vi "Pelletron_Conditioning.vi"(6 "Desired Voltage (MV)":dbl, 7 "Condition Start time":dbl, 8 "error in (no error)":errorcluster, 9 "Input Old Cluster":T1, 10 "Input New Cluster":T2, 11 "AccelNET.lvlib:TCP.lvclass":refnum<class "TCP.lvclass">) -> (0 "Error Out":errorcluster, 1 "Conditioning?":bool, 2 "Step Up Voltage?":bool)   [LabVIEW 2012, in "AccelNET.lvlib" / "TCP.lvclass"]
uses:
  TCP.lvclass
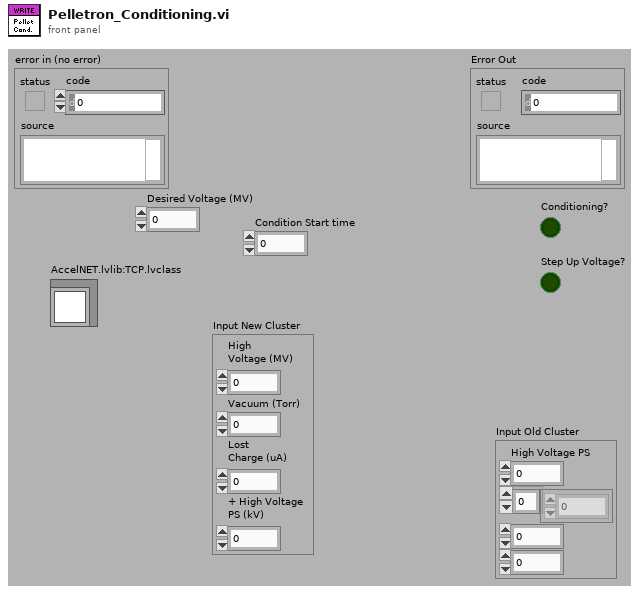
[diagram p1: front panel]
types:
  T1 = cluster{"High Voltage PS":dbl, "Pressure":dbl[], "Lost Charge":dbl, "High Voltage":dbl}
  T2 = cluster{"High\nVoltage (MV)":dbl, "Vacuum (Torr)":dbl, "Lost\nCharge (uA)":dbl, "+ High Voltage\nPS (kV)":dbl}
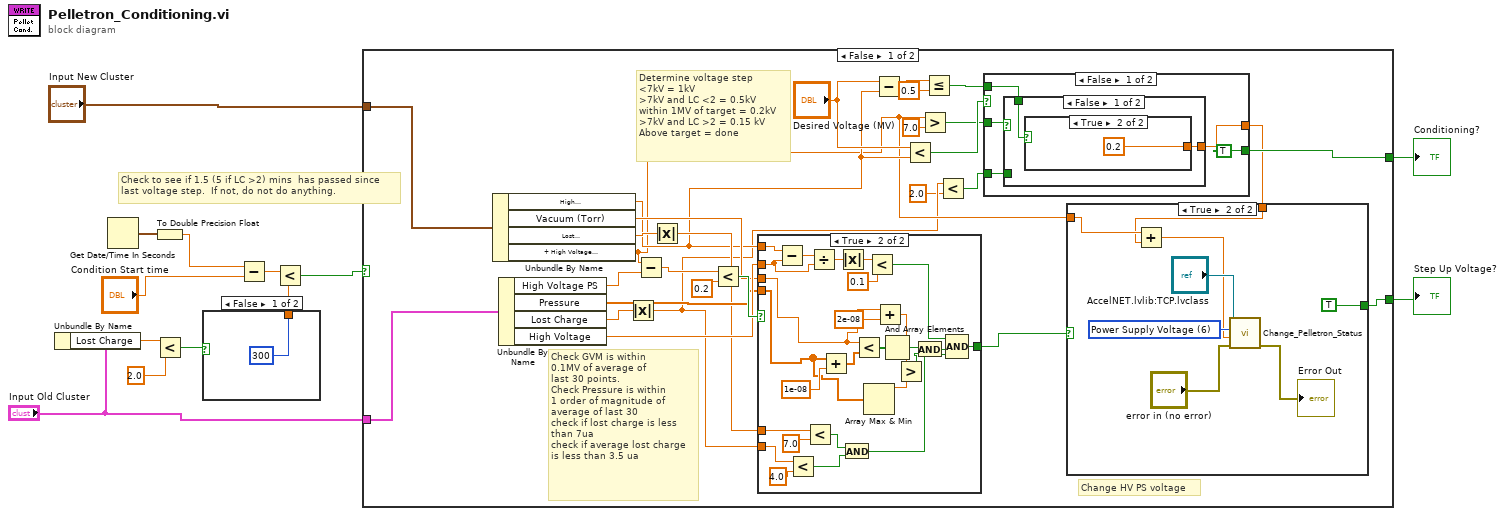
[diagram p0: block diagram]
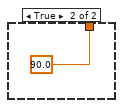
[diagram p2: hidden frame]
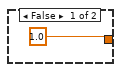
[diagram p3: hidden frame]
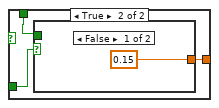
[diagram p4: hidden frame]
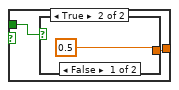
[diagram p5: hidden frame]
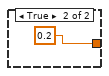
[diagram p6: hidden frame]
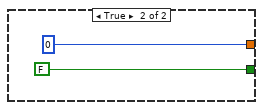
[diagram p7: hidden frame]
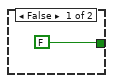
[diagram p8: hidden frame]
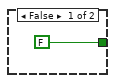
[diagram p9: hidden frame]
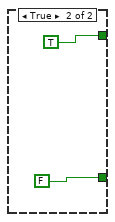
[diagram p10: hidden frame]
diagram:
  # "Check to see if 1.5 (5 if LC >2) mins  has passed since\nlast voltage step.  If not, do not do anything."
  n1 = Unbundle By Name("Input Old Cluster") -> ("Lost Charge"=w3:dbl)
  n2 = Get Date/Time In Seconds() -> (seconds since 1Jan1904=w13:timestamp)
  n3 = To Double Precision Float(number=w13) -> (double precision float=w12:dbl)
  n4 = Less?(x=w3, y=2.0) -> (x < y?=w1:bool)
  n5 = case shown="False" w1 {
    tunnel: [300 90.0 ("y")] -> w9
    frame False {
    }
    frame True {
    }
  }
  n6 = Subtract(x=w12, y="Condition Start time") -> (x-y=w10:dbl)
  n7 = Less?(x=w10, y=w9) -> (x < y?=w8:bool)
  n8 = case shown="False" w8 {
    tunnel: [w28 FALSE] -> w7
    tunnel: [w27 TRUE] -> w6
    tunnel: "Input New Cluster" -> [w20 _]
    tunnel: "Input Old Cluster" -> [w19 _]
    frame False {
      # "Change HV PS voltage"
      # "Determine voltage step\n<7kV = 1kV\n>7kV and LC <2 = 0.5kV\nwithin 1MV of target = 0.2kV\n>7kV and LC >2 = 0.15 kV\nAbove target = done"
      # "Check GVM is within\n0.1MV of average of\nlast 30 points.\nCheck Pressure is within\n1 order of magnitude of\naverage of last 30\ncheck if lost charge is less\nthan 7ua\ncheck if average lost charge\nis less than 3.5 ua"
      n9 = Unbundle By Name(w20) -> ("High\nVoltage (MV)"=w26:dbl, "Vacuum (Torr)"=w39:dbl, "Lost\nCharge (uA)"=w37:dbl, "+ High Voltage\nPS (kV)"=w21:dbl)
      n10 = Unbundle By Name(w19) -> ("High Voltage PS"=w43:dbl, "Pressure"=w38:dbl[], "Lost Charge"=w36:dbl, "High Voltage"=w40:dbl)
      n11 = Absolute Value(x=w36) -> (abs(x)=w18:dbl)
      n12 = Subtract(x=w21, y=w43) -> (x-y=w22:dbl)
      n13 = Absolute Value(x=w37) -> (abs(x)=w35:dbl)
      n14 = Less?(x=w22, y=0.2) -> (x < y?=w41:bool)
      n15 = case shown="True" w41 {
        tunnel: w26 -> [_ w94]
        tunnel: w40 -> [_ w92]
        tunnel: w39 -> [_ w76]
        tunnel: w38 -> [_ w80]
        tunnel: w35 -> [_ w98]
        tunnel: w18 -> [_ w96]
        tunnel: [FALSE w85] -> w23
        frame False {
        }
        frame True {
          n16 = Subtract(x=w94, y=w92) -> (x-y=w93:dbl)
          n17 = Less?(x=w96, y=4.0) -> (x < y?=w88:bool)
          n18 = Less?(x=w98, y=7.0) -> (x < y?=w89:bool)
          n19 = Divide(x=w93, y=w92) -> (x/y=w91:dbl)
          n20 = Add(x=w80, y=1e-08) -> (x+y=w81:dbl[])
          n21 = Absolute Value(x=w91) -> (abs(x)=w83:dbl)
          n22 = And(x=w89, y=w88) -> (x .and. y?=w86:bool)
          n23 = Less?(x=w76, y=w81) -> (x < y?=w84:bool[])
          n24 = Array Max & Min(array=w80) -> (max value=w78:dbl)  [unwired: 3 out]
          n25 = Less?(x=w83, y=0.1) -> (x < y?=w87:bool)
          n26 = Add(x=w76, y=2e-08) -> (x+y=w74:dbl)
          n27 = And Array Elements(Boolean array=w84) -> (logical AND=w79:bool)
          n28 = Greater?(x=w74, y=w78) -> (0:w77:bool)
          n29 = And(x=w79, y=w77) -> (x .and. y?=w73:bool)
          n30 = Compound Arithmetic op=AND(w87, w73, w86) -> (w85:bool)
        }
      }
      n31 = Subtract(x="Desired Voltage (MV)", y=w26) -> (x-y=w33:dbl)
      n32 = Less?(x="Desired Voltage (MV)", y=w26) -> (x < y?=w30:bool)
      n33 = Greater?(x=w21, y=7.0) -> (0:w25:bool)
      n34 = Less Or Equal?(x=w33, y=0.5) -> (x <= y?=w29:bool)
      n35 = Less?(x=w18, y=2.0) -> (x < y?=w16:bool)
      n36 = case shown="False" w30 {
        tunnel: [TRUE FALSE] -> w27
        tunnel: [w45 0] -> w24
        tunnel: w29 -> [w47 _]
        tunnel: w25 -> [w48 _]
        tunnel: w16 -> [w44 _]
        frame False {
          n37 = case shown="False" w48 {
            tunnel: w47 -> [w50 w55]
            tunnel: [w49 w54] -> w45
            tunnel: w44 -> [_ w53]
            frame False {
              n38 = case shown="True" w50 {
                tunnel: [1.0 ("y") 0.2 ("y")] -> w49
                frame False {
                }
                frame True {
                }
              }
            }
            frame True {
              n39 = case shown="False" w53 {
                tunnel: w55 -> [_ w58]
                tunnel: [0.15 w57] -> w54
                frame False {
                }
                frame True {
                  n40 = case shown="False" w58 {
                    tunnel: [0.5 ("y") 0.2 ("y")] -> w57
                    frame False {
                    }
                    frame True {
                    }
                  }
                }
              }
            }
          }
        }
        frame True {
        }
      }
      n41 = case shown="True" w23 {
        tunnel: [FALSE TRUE] -> w28
        tunnel: w24 -> [_ w65]
        tunnel: w21 -> [_ w66]
        frame False {
        }
        frame True {
          w71 = u16 6 items=["GV", "Blower", "Main Power Supply", "Chain Power Supply", "Chain", "Rotating Shaft", "Power Supply Voltage", "Control Mode", "Control Mode Reference", "Chain Bypass", "Rotating Shaft Bypass", "Spark Counter", "Spark Limit", "Threshold", "Spark Counter Reset", "Ion Filament"] ("Write Selector")
          n42 = Add(x=w66, y=w65) -> (x+y=w64:dbl)
          n43 = call "Change_Pelletron_Status.vi"("error in (no error)"="error in (no error)", "Write Value"=w64, "Write Selector"=w71, "AccelNET.lvlib:TCP.lvclass"="AccelNET.lvlib:TCP.lvclass") -> ("error out"=→"Error Out":errorcluster)  [unwired: 7 in]
        }
      }
    }
    frame True {
    }
  }
  "Step Up Voltage?" <- w7
  "Conditioning?" <- w6
